vi "Laurel Modbus Read Rate and Total.vi"(8 "error in (no error)":errorcluster, 11 "Modbus Master in":refnum<class "Modbus Master.lvclass">) -> (0 "error out":errorcluster, 1 "Totalizer":dbl, 2 "Rate":dbl, 3 "Modbus Master out":refnum<class "Modbus Master.lvclass">)   [LabVIEW 2020]
uses:
  <vilib>/NI/Modbus Library/API/Master/Modbus Master.lvclass
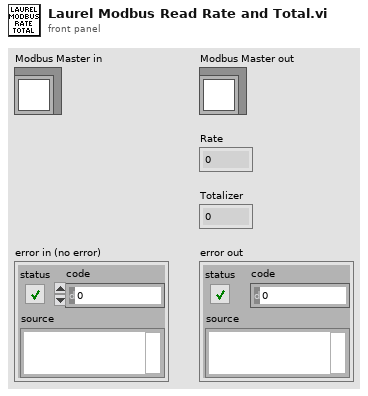
[diagram p1: front panel]
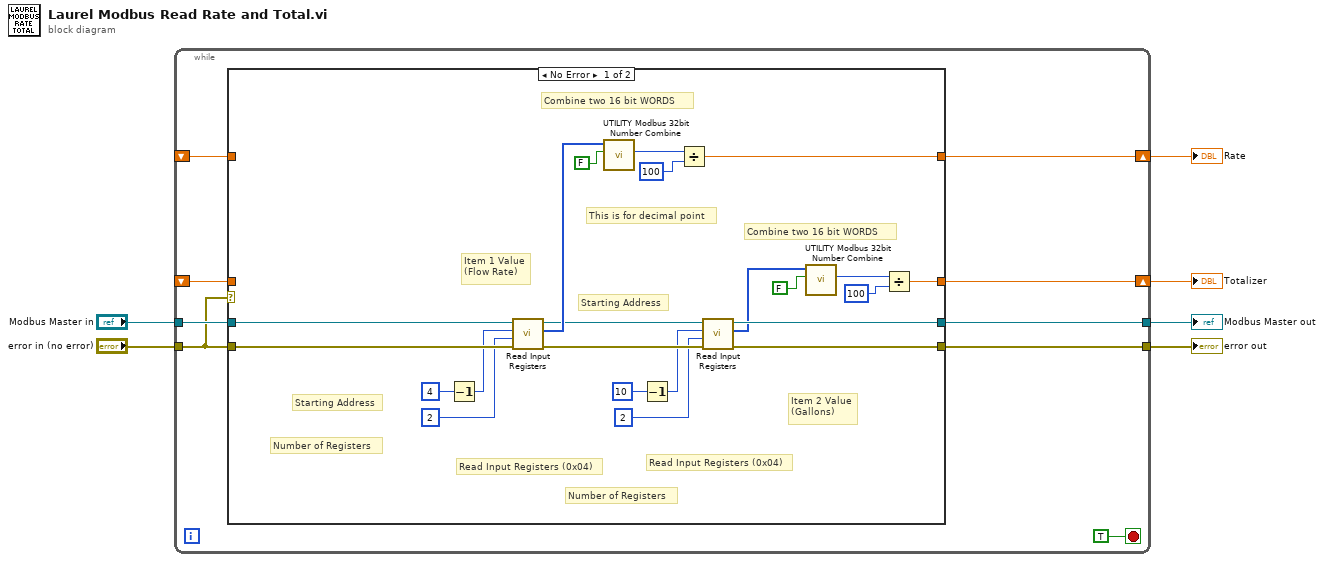
[diagram p0: block diagram]
diagram:
  n1 = while {
    tunnel: "error in (no error)" -> [w10]
    tunnel: [w14] -> w4
    tunnel: "Modbus Master in" -> [w15]
    tunnel: [w13] -> w3
    shift-right: [w12] -> w1
    shift-left: _ -> [w9]
    shift-right: [w11] -> w2
    shift-left: _ -> [w8]
    stop <- TRUE stop-if-true
    n2 = case shown="No Error" w10 {
      tunnel: w10 -> [w37 w38]
      tunnel: w15 -> [w36 w39]
      tunnel: [w35 w38] -> w14
      tunnel: [w34 w39] -> w13
      tunnel: [w17 w41] -> w12
      tunnel: [w16 w40] -> w11
      tunnel: w9 -> [_ w41]
      tunnel: w8 -> [_ w40]
      frame No Error {
        # "Combine two 16 bit WORDS"
        # "Starting Address"
        # "Number of Registers"
        # "Read Input Registers (0x04)"
        # "Item 2 Value\n(Gallons)"
        # "This is for decimal point"
        # "Combine two 16 bit WORDS"
        # "Starting Address"
        # "Number of Registers"
        # "Read Input Registers (0x04)"
        # "Item 1 Value\n(Flow Rate)"
        n3 = Decrement(x=u16 4 ("starting address 2")) -> (x-1=w26:u16)
        n4 = call-dynamic "Read Input Registers.vi"("error in"=w37, "number of inputs"=u16 2, "starting address"=w26, "Modbus master in"=w36) -> ("error out"=w33:errorcluster, "register values"=w29:u16[], "Modbus master out"=w27:refnum<class "Modbus Master.lvclass">)  [unwired: 5 in]
        n5 = call "UTILITY Modbus 32bit Number Combine.vi"("Swap Words"=FALSE, "Holding Registers"=w29) -> ("word swapped"=w31:u32)  [unwired: 8 in, 1 out]
        n6 = Decrement(x=u16 10 ("starting address 2")) -> (x-1=w18:u16)
        n7 = Divide(x=w31, y=u32 100) -> (x/y=w17:dbl)
        n8 = call-dynamic "Read Input Registers.vi"("error in"=w33, "number of inputs"=u16 2, "starting address"=w18, "Modbus master in"=w27) -> ("error out"=w35:errorcluster, "register values"=w21:u16[], "Modbus master out"=w34:refnum<class "Modbus Master.lvclass">)  [unwired: 5 in]
        n9 = call "UTILITY Modbus 32bit Number Combine.vi"("Swap Words"=FALSE, "Holding Registers"=w21) -> ("word swapped"=w23:u32)  [unwired: 8 in, 1 out]
        n10 = Divide(x=w23, y=u32 100) -> (x/y=w16:dbl)
      }
      frame Error {
      }
    }
  }
  "error out" <- w4
  "Modbus Master out" <- w3
  "Totalizer" <- w2
  "Rate" <- w1
